vi "Drive_getAbortPositionControl.vi"(8 "error in (no error)":errorcluster) -> (0 "error out":errorcluster, 2 "Abort Position Control":bool)   [LabVIEW 2009, in "Drive.lvlib"]
uses:
  Drive.lvlib
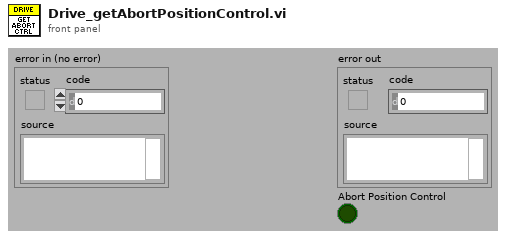
[diagram p1: front panel]
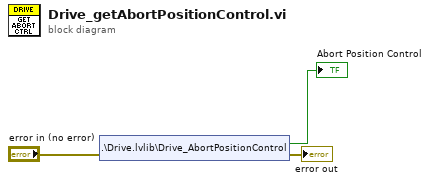
[diagram p0: block diagram]
diagram:
  n1 = shared-variable ".\\Drive.lvlib\\Drive_AbortPositionControl"(error in="error in (no error)") -> (→"Abort Position Control":bool, error out=→"error out":errorcluster)
